vi "TimeInterpVariant_New.vi"(11 "MaxTime":dbl=1.0) -> (3 "TimeInterpVariant":T1)   [LabVIEW 2019, in "Trajectory_Library.lvlib"]
doc: "Create the data cluster for a TIME_INTERPOLATABLE_VARIANT\n\nThe TimeInterpolatableVariant provides an easy way to estimate past measurements. One application might be in conjunction with the DifferentialDrivePoseEstimator, where knowledge of the robot pose at the time when vision or other global measurement were recorded is necessary, or for recording the past angles of mechanisms as measured by encoders.\n\nThe TIME_INTERPOLATABLE_VARIANT stores and returns Variant values. Because this routine stores and retrieves Variant values, several custom routines will need to be provided to effectively use this set of functions:\n -- A TypeDef for the cluster containing the data to be sotred.\n -- A routine to pack data into the custom TypeDef\n -- A routine to unpack the variant data back to the custom data type.\n -- A routine to interpolate two values. A sample routine, \n TimeInterpVariant_Interpolate.vi, is provided to use as a template \n to create the custom interpolation routine.\n\nInputs:\n - Max Time -- The maximum time (seconds) of data to store in the buffer.\n\nOutputs:\n - Time InterpVariant -- Created data structure cluster"
uses:
  Trajectory_Library.lvlib
  TypeDef/TIME_INTERPOLATABLE_VARIANT.ctl
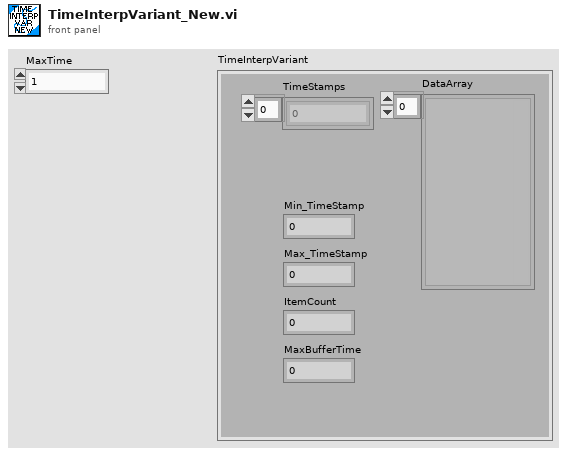
[diagram p1: front panel]
types:
  T1 = typedef "Trajectory_Library.lvlib/TIME_INTERPOLATABLE_VARIANT.ctl" = cluster{"TimeStamps":dbl[], "DataArray":variant[], "Min_TimeStamp":dbl, "Max_TimeStamp":dbl, "ItemCount":i32, "MaxBufferTime":dbl}
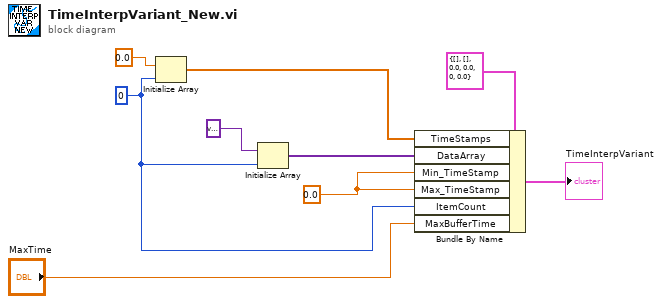
[diagram p0: block diagram]
diagram:
  w6 = 0.0 ("X")
  w3 = 0 ("dimension size")
  n1 = Initialize Array(0.0 ("element"), w3) -> (w7:dbl[])
  n2 = Initialize Array(variant, w3) -> (w4:variant[])
  n3 = Bundle By Name(cluster=T1 {"TimeStamps"=[], "DataArray"=[], "Min_TimeStamp"=0.0, "Max_TimeStamp"=0.0, "ItemCount"=0, "MaxBufferTime"=0.0} ("TIME_INTERPOLATABLE_POSE"), "TimeStamps"=w7, "DataArray"=w4, "Min_TimeStamp"=w6, "Max_TimeStamp"=w6, "ItemCount"=w3, "MaxBufferTime"="MaxTime") -> (→"TimeInterpVariant":T1)
